vi "写入Source.vi"(8 "error in (no error)":errorcluster caption="错误输入（无错误）", 10 "Source":cluster{"X":dbl, "Y":dbl}, 11 "Navigation输入":refnum<class "Navigation.lvclass">) -> (0 "error out":errorcluster caption="错误输出", 3 "Navigation输出":refnum<class "Navigation.lvclass">)   [LabVIEW 2018, in "Navigation.lvclass"]
uses:
  Navigation.lvclass
  Navigation.lvclass/Navigation.ctl
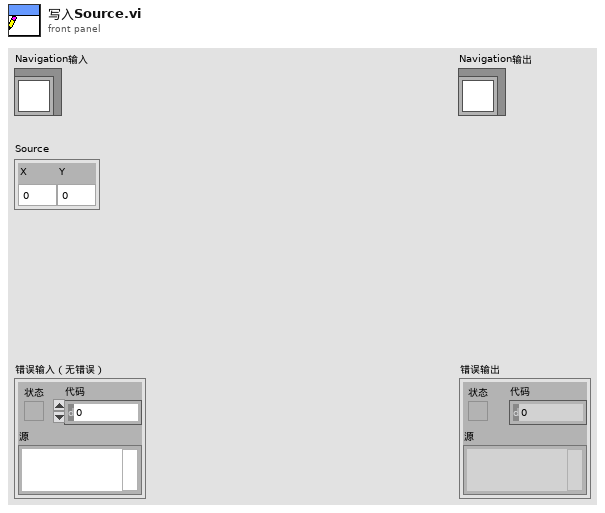
[diagram p1: front panel]
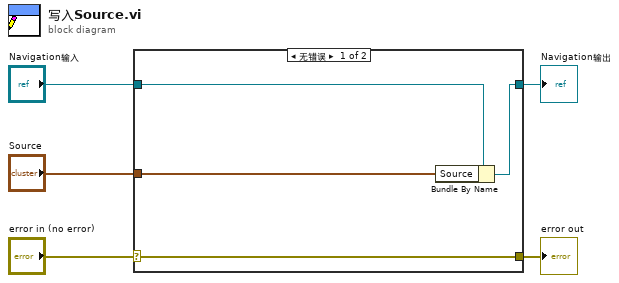
[diagram p0: block diagram]
diagram:
  n1 = case shown="无错误" "error in (no error)" {
    selector: "error in (no error)" -> [w9 w10]
    tunnel: [w9 w10] -> w4
    tunnel: [w7 w11] -> w2
    tunnel: "Navigation输入" -> [w8 w11]
    tunnel: "Source" -> [w6 _]
    frame No Error {
      n2 = Bundle By Name(cluster=w8, "Source"=w6) -> (w7:refnum<class "Navigation.lvclass">)
    }
    frame Error {
    }
  }
  "error out" <- w4
  "Navigation输出" <- w2
